vi "数采仪日志报警存储(子VI).vi"   [LabVIEW 2016]
types:
  T1 = cluster{"时间标识":timestamp, "设备":string, "日志信息":string, "流程参数":string}
  T2 = cluster{"时间标识":timestamp, "设备":string, "日志信息":string}
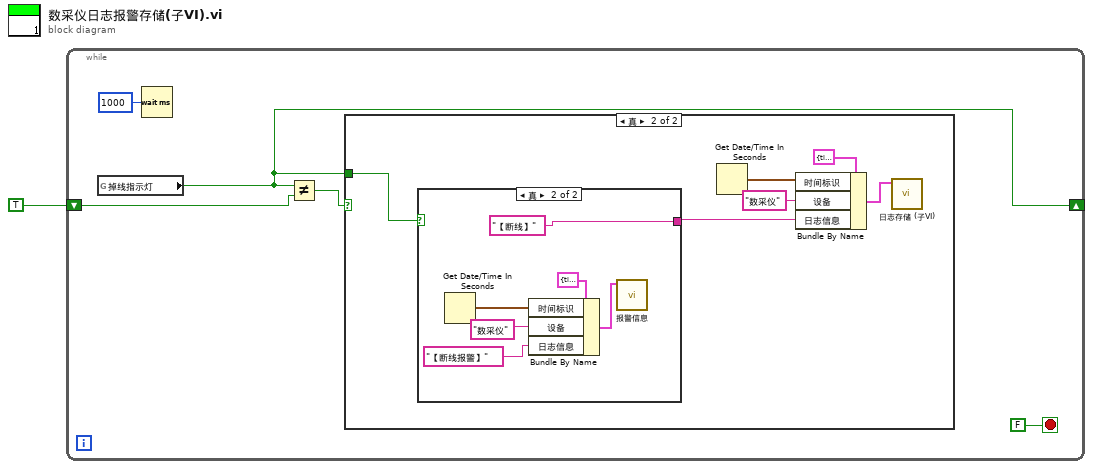
[diagram p0: block diagram]
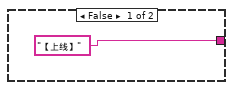
[diagram p3: hidden frame]
diagram:
  n1 = while {
    shift-right: [w2] -> _
    shift-left: TRUE -> [w3]
    stop <- FALSE stop-if-true
    n2 = global read "全局 数据发送重叠.vi" "掉线指示灯"() -> (w2:bool)
    n3 = Wait (ms)(milliseconds to wait=u32 1000 ("等待时间（毫秒）")) -> ()  [unwired: 1 out]
    n4 = Not Equal?(x=w2, y=w3) -> (x != y?=w4:bool)
    n5 = case shown="真" w4 {
      tunnel: w2 -> [_ w7]
      frame False {
      }
      frame True {
        n6 = case shown="真" w7 {
          tunnel: ["【上线】" ("设备") "【断线】" ("设备")] -> w8
          frame False {
          }
          frame True {
            n7 = Get Date/Time In Seconds() -> (seconds since 1Jan1904=w16:timestamp)
            n8 = Bundle By Name(cluster=T2 {"时间标识"=timestamp(0 s since 1904-01-01), "设备"="", "日志信息"=""} ("data in"), "时间标识"=w16, "设备"="数采仪", "日志信息"="【断线报警】" ("设备")) -> (w17:T2)
            n9 = call "报警信息.vi"("data in"=w17) -> ()  [unwired: 10 in, 1 out]
          }
        }
        n10 = Get Date/Time In Seconds() -> (seconds since 1Jan1904=w10:timestamp)
        n11 = Bundle By Name(cluster=T1 {"时间标识"=timestamp(0 s since 1904-01-01), "设备"="", "日志信息"="", "流程参数"=""} ("data in"), "时间标识"=w10, "设备"="数采仪", "日志信息"=w8) -> (w11:T1)
        n12 = call "日志存储 (子VI).vi"("data in"=w11) -> ()  [unwired: 11 in]
      }
    }
  }
